vi "doTesting.vi"() -> ()   [LabVIEW 2009, in "run.lvlib"]
uses:
  run.lvlib
  Channels/Digital/DigitalOutput.lvclass
  Channels/VoltOutput/AnalogOutput.lvclass
panel:
  in  "Data":T1={"Timestamps ms"=[0.0, 1000.0, 2000.0, 3000.0, 4000.0, 5000.0], "Camera"=[0, 0, 1, 1, 1, 0], "AnalogData"=[[1, 0, 1, 1], [1, 0, 1, 1], [0, 1, 0, 0], [0, 1, 0, 0], [0, 1, 0, 0], [0, 0, 0, 0]], "AnalogChannels"=["Aom2", "Aom3", "Bottom Coil", "Top Coil", "Camera"], "Aom2 Amp Volts"=0.863, "Aom3 Amp Volts"=0.07, "BottomCoil Volts"=0.96, "TopCoil Volts"=0.76, "Trigger Pulse Length ms"=0.001} {"AnalogData" items=["On"=1, "Off"=0]; "Camera" items=["On"=1, "Off"=0, "Init"=2]; "Timestamps ms" format="%#_10g"}
  in  "stop":bool
  # "Stop Acquisition Before\nits finished."
  # "Analog Output Channels ao0 to ao3"
  # "Digital Port0 Line1"
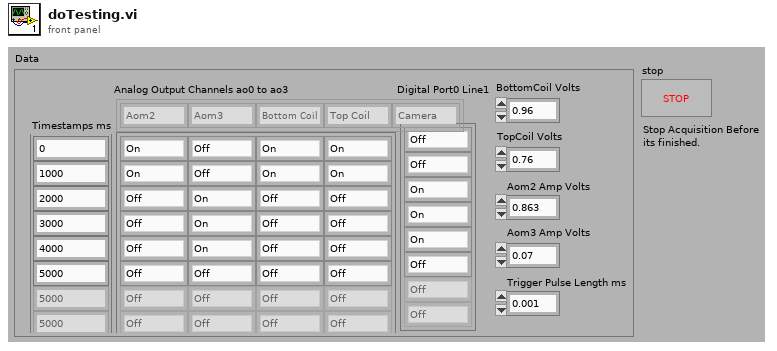
[diagram p1: front panel]
types:
  T1 = cluster{"Timestamps ms":dbl[], "Camera":u16[], "AnalogData":u16[][], "AnalogChannels":string[], "Aom2 Amp Volts":dbl, "Aom3 Amp Volts":dbl, "BottomCoil Volts":dbl, "TopCoil Volts":dbl, "Trigger Pulse Length ms":dbl}
  T2 = cluster{"Name":string, "Channels":string, "Ranges":dbl[]}
  T3 = cluster{"Clock source":string, "Clock rate":dbl, "Start trigger line":string, "Sample Rate":dbl, dbl}
  T4 = cluster{"Master Clock source":string, "Master Clock rate":dbl, "Start trigger line":string, "Scan rate":dbl, "Stop trigger line":string, dbl}
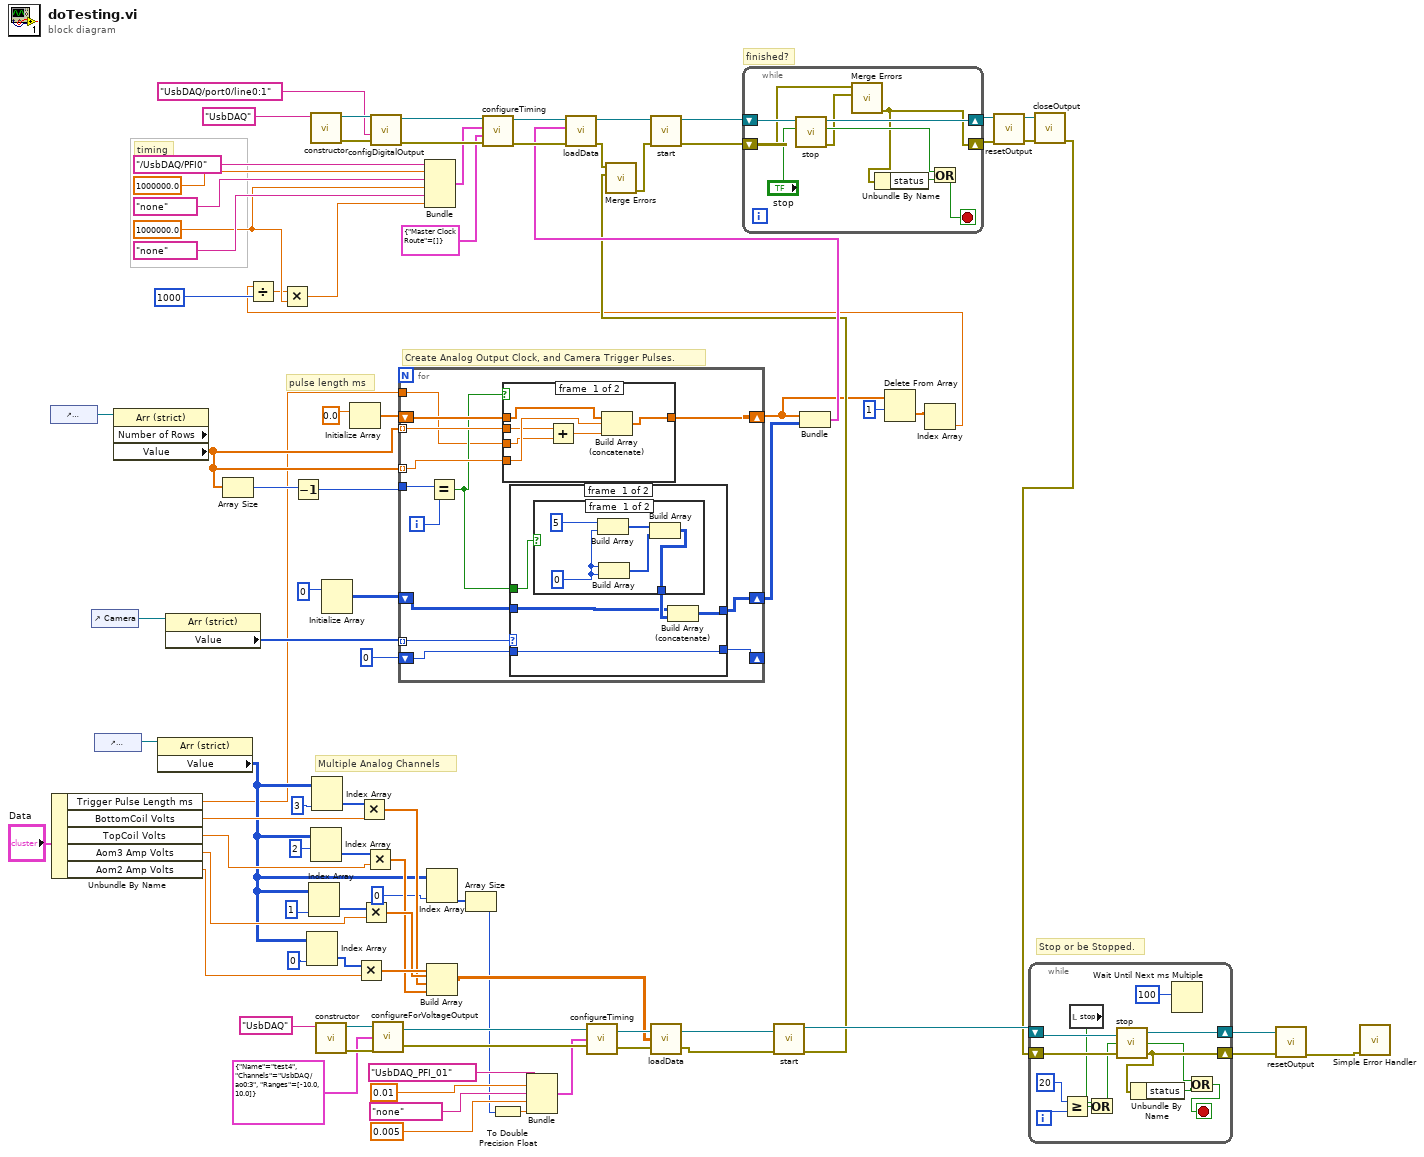
[diagram p0: block diagram]
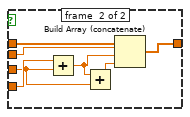
[diagram p2: hidden frame]
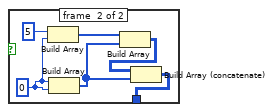
[diagram p3: hidden frame]
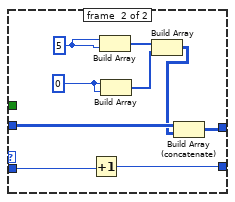
[diagram p4: hidden frame]
diagram:
  w62 = 1000000.0 ("Scan rate")
  # "pulse length ms"
  # "finished?"
  # "Stop or be Stopped."
  # "Multiple Analog Channels"
  # "Create Analog Output Clock, and Camera Trigger Pulses."
  # "timing"
  n1 = control-ref of="Timestamps ms"() -> (w73:refnum<vi>)
  n2 = Unbundle By Name("Data") -> ("Trigger Pulse Length ms"=w9:dbl, "BottomCoil Volts"=w24:dbl, "TopCoil Volts"=w23:dbl, "Aom3 Amp Volts"=w22:dbl, "Aom2 Amp Volts"=w21:dbl)
  n3 = control-ref of="Camera"() -> (w71:refnum<vi>)
  n4 = control-ref of="AnalogData"() -> (w57:refnum<vi>)
  n5 = property class="Arr (strict)" props=["Number of Rows", "Value"](reference=w73) -> ("Value"=w61:dbl[])  [unwired: 1 in, 3 out]
  n6 = property class="Arr (strict)"(reference=w57) -> ("Value"=w18:u16[][])  [unwired: 1 in, 2 out]
  n7 = property class="Arr (strict)"(reference=w71) -> ("Value"=w64:u16[])  [unwired: 1 in, 2 out]
  n8 = Array Size(array=w61) -> (size(s)=w63:i32)
  n9 = Decrement(x=w63) -> (x-1=w58:i32)
  n10 = Index Array(array=w18, index (col)=0) -> (element=w45:u16[])  [unwired: 1 in]
  n11 = Index Array(array=w18, index (col)=1) -> (element=w53:u16[])  [unwired: 1 in]
  n12 = call "constructor.vi"("deviceName"="UsbDAQ") -> ("error out"=w76:errorcluster, "DigitalOutput out"=w77:refnum<class "DigitalOutput.lvclass">)  [unwired: 9 in]
  n13 = Index Array(array=w18, index (col)=2) -> (element=w51:u16[])  [unwired: 1 in]
  n14 = Index Array(array=w18, index (col)=3) -> (element=w49:u16[])  [unwired: 1 in]
  n15 = call "constructor.vi"("deviceName"="UsbDAQ") -> ("error out"=w37:errorcluster, "AnalogOutput out"=w38:refnum<class "AnalogOutput.lvclass">)  [unwired: 9 in]
  n16 = Initialize Array(0) -> (w67:i32[][])  [unwired: 2 in]
  n17 = Initialize Array(0.0) -> (w70:dbl[])  [unwired: 1 in]
  n18 = Multiply(x=w45, y=w21) -> (x*y=w55:dbl[])
  n19 = Multiply(x=w49, y=w24) -> (x*y=w47:dbl[])
  n20 = Multiply(x=w53, y=w22) -> (x*y=w50:dbl[])
  n21 = Multiply(x=w51, y=w23) -> (x*y=w46:dbl[])
  n22 = call-dynamic "configDigitalOutput.vi"("error in (no error)"=w76, "Physical Channels"="UsbDAQ/port0/line0:1", "DigitalOutput in"=w77) -> ("error out"=w89:errorcluster, "DigitalOutput out"=w90:refnum<class "DigitalOutput.lvclass">)  [unwired: 7 in]
  n23 = call-dynamic "configureForVoltageOutput.vi"("error in (no error)"=w37, "Output Properties"=T2 {"Name"="test4", "Channels"="UsbDAQ/ao0:3", "Ranges"=[-10.0, 10.0]}, "AnalogOutput in"=w38) -> ("error out"=w43:errorcluster, "AnalogOutput out"=w44:refnum<class "AnalogOutput.lvclass">)
  n24 = for {
    shift-right: [w99] -> w69
    shift-left: w67 -> [w100]
    tunnel: w61 -> [w103] mode=indexing
    shift-right: [w102] -> w14
    shift-left: w70 -> [w101]
    tunnel: w61 -> [w98] mode=indexing
    tunnel: w64 -> [w97] mode=indexing
    shift-right: [w95] -> _
    shift-left: 0 -> [w96]
    tunnel: w58 -> [w94]
    tunnel: w9 -> [w91]
    i -> [w93]
    n25 = Equal?(x=w94, y=w93) -> (x = y?=w92:bool)
    n26 = case shown="True" w92 {
      tunnel: w103 -> [w109 w113]
      tunnel: [w107 w115] -> w102
      tunnel: w101 -> [w106 w116]
      tunnel: w98 -> [w105 w114]
      tunnel: w91 -> [w104 w110]
      frame #0 {
        n27 = Add(x=w105, y=w104) -> (x+y=w108:dbl)
        n28 = Build Array (concatenate)(w106, w109, w108) -> (w107:dbl[])
      }
      frame #1 {
        n29 = Add(x=w113, y=w110) -> (x+y=w112:dbl)
        n30 = Add(x=w112, y=w110) -> (x+y=w111:dbl)
        n31 = Build Array (concatenate)(w116, w114, w112, w111) -> (w115:dbl[])
      }
    }
    n32 = case shown="0, Default" w97 {
      tunnel: w100 -> [w120 w141]
      tunnel: [w119 w140] -> w99
      tunnel: w96 -> [w118 w138]
      tunnel: [w118 w137] -> w95
      tunnel: w92 -> [w117 _]
      frame #0 {
        n33 = case shown="True" w117 {
          tunnel: [w126 w129] -> w121
          frame #0 {
            w122 = 0
            n34 = Build Array(5, w122) -> (w125:i32[])
            n35 = Build Array(w122, w122) -> (w124:i32[])
            n36 = Build Array(w125, w124) -> (w126:i32[][])
          }
          frame #1 {
            w130 = 0
            n37 = Build Array(5, w130) -> (w132:i32[])
            n38 = Build Array(w130, w130) -> (w127:i32[])
            n39 = Build Array(w132, w127) -> (w128:i32[][])
            n40 = Build Array (concatenate)(w128, w127) -> (w129:i32[][])
          }
        }
        n41 = Build Array (concatenate)(w120, w121) -> (w119:i32[][])
      }
      frame #1 {
        w133 = 0
        w134 = 5
        n42 = Increment(x=w138) -> (x+1=w137:i32)
        n43 = Build Array(w134, w134) -> (w136:i32[])
        n44 = Build Array(w133, w133) -> (w135:i32[])
        n45 = Build Array(w136, w135) -> (w139:i32[][])
        n46 = Build Array (concatenate)(w141, w139) -> (w140:i32[][])
      }
    }
  }
  n47 = Index Array(array=w18, index (col)=0) -> (element=w19:u16[])  [unwired: 1 in]
  n48 = Build Array(w55, w50, w47, w46) -> (w17:dbl[][])
  n49 = Array Size(array=w19) -> (size(s)=w10:i32)
  n50 = To Double Precision Float(number=w10) -> (double precision float=w29:dbl)
  n51 = Bundle("Clock source"="UsbDAQ_PFI_01", "Clock rate"=0.01, "Start trigger line"="none", "Sample Rate"=0.005, w29) -> (w34:T3)  [unwired: 1 in]
  n52 = call-dynamic "configureTiming.vi"("error in (no error)"=w43, "Timing"=w34, "AnalogOutput in"=w44) -> ("error out"=w41:errorcluster, "AnalogOutput out"=w42:refnum<class "AnalogOutput.lvclass">)
  n53 = call-dynamic "loadData.vi"("error in (no error)"=w41, "Data"=w17, "AnalogOutput in"=w42) -> ("error out"=w39:errorcluster, "AnalogOutput out"=w40:refnum<class "AnalogOutput.lvclass">)
  n54 = call-dynamic "start.vi"("error in (no error)"=w39, "AnalogOutput in"=w40) -> ("error out"=w25:errorcluster, "AnalogOutput out"=w28:refnum<class "AnalogOutput.lvclass">)  [unwired: 8 in]
  n55 = Bundle(w14, w69) -> (w65:cluster{dbl[], i32[][]})  [unwired: 1 in]
  n56 = Delete From Array(array=w14, length=1) -> (deleted portion=w12:dbl[])  [unwired: 1 in, 1 out]
  n57 = Index Array(array=w12) -> (element=w11:dbl)  [unwired: 1 in]
  n58 = Divide(x=w11, y=1000) -> (x/y=w60:dbl)
  n59 = Multiply(x=w60, y=w62) -> (x*y=w15:dbl)
  n60 = Bundle("Master Clock source"="/UsbDAQ/PFI0", "Master Clock rate"=1000000.0, "Start trigger line"="none", "Scan rate"=w62, "Stop trigger line"="none", w15) -> (w80:T4)  [unwired: 1 in]
  n61 = call-dynamic "configureTiming.vi"("error in (no error)"=w89, "Routings"=cluster{"Master Clock Route":string[]} {"Master Clock Route"=[]}, "Timing"=w80, "DigitalOutput in"=w90) -> ("error out"=w87:errorcluster, "DigitalOutput out"=w88:refnum<class "DigitalOutput.lvclass">)  [unwired: 6 in]
  n62 = call-dynamic "loadData.vi"("error in (no error)"=w87, "Data"=w65, "DigitalOutput in"=w88) -> ("error out"=w27:errorcluster, "DigitalOutput out"=w86:refnum<class "DigitalOutput.lvclass">)  [unwired: 7 in]
  n63 = call <vilib>:"Merge Errors.vi"("error in 2 (no error)"=w25, "error in 1 (no error)"=w27) -> ("error out"=w26:errorcluster)  [unwired: 5 in]
  n64 = call-dynamic "start.vi"("error in (no error)"=w26, "DigitalOutput in"=w86) -> ("error out"=w78:errorcluster, "DigitalOutput out"=w85:refnum<class "DigitalOutput.lvclass">)  [unwired: 8 in]
  n65 = while {
    shift-right: [w149] -> w7
    shift-left: w85 -> [w150]
    shift-right: [w142] -> w4
    shift-left: w78 -> [w144]
    stop <- w146 stop-if-true
    n66 = call-dynamic "stop.vi"("stop"="stop", "DigitalOutput in"=w150) -> ("error out"=w143:errorcluster, "stopped"=w148:bool, "DigitalOutput out"=w149:refnum<class "DigitalOutput.lvclass">)  [unwired: 7 in]
    n67 = call <vilib>:"Merge Errors.vi"("error in 2 (no error)"=w143, "error in 1 (no error)"=w144) -> ("error out"=w142:errorcluster)  [unwired: 5 in]
    n68 = Unbundle By Name(w142) -> ("status"=w147:bool)
    n69 = Or(x=w148, y=w147) -> (x .or. y?=w146:bool)
  }
  n70 = call-dynamic "resetOutput.vi"("error in (no error)"=w4, "DigitalOutput in"=w7) -> ("error out"=w5:errorcluster, "DigitalOutput out"=w6:refnum<class "DigitalOutput.lvclass">)  [unwired: 8 in]
  n71 = call-dynamic "closeOutput.vi"("error in (no error)"=w5, "DigitalOutput in"=w6) -> ("error out"=w8:errorcluster)  [unwired: 9 in]
  n72 = while {
    shift-right: [w161] -> w2
    shift-left: w28 -> [w162]
    shift-right: [w160] -> w3
    shift-left: w8 -> [w163]
    i -> [w155]
    stop <- w158 stop-if-true
    n73 = Greater Or Equal?(x=20, y=w155) -> (x >= y?=w154:bool)
    n74 = local read "stop"() -> (w152:bool)
    n75 = Or(x=w152, y=w154) -> (x .or. y?=w151:bool)
    n76 = call-dynamic "stop.vi"("error in (no error)"=w163, "stop"=w151, "AnalogOutput in"=w162) -> ("error out"=w160:errorcluster, "Stopped"=w159:bool, "AnalogOutput out"=w161:refnum<class "AnalogOutput.lvclass">)
    n77 = Unbundle By Name(w160) -> ("status"=w153:bool)
    n78 = Wait Until Next ms Multiple(millisecond multiple=100) -> ()  [unwired: 1 out]
    n79 = Or(x=w159, y=w153) -> (x .or. y?=w158:bool)
  }
  n80 = call-dynamic "resetOutput.vi"("error in (no error)"=w3, "AnalogOutput in"=w2) -> ("error out"=w1:errorcluster)  [unwired: 8 in, 1 out]
  n81 = call <vilib>:"Simple Error Handler.vi"("error in (no error)"=w1) -> ()  [unwired: 4 in, 5 out]
